vi "ex_3_testy.vi"() -> ()   [LabVIEW 2020]
panel:
  out "XY Graph 4":cluster{i32[], i32[]}(graph)
  out "XY Graph 3":cluster{i32[], i32[]}(graph)
  out "XY Graph 2":cluster{i32[], i32[]}(graph)
  out "XY Graph":cluster{i32[], i32[]}[](graph)
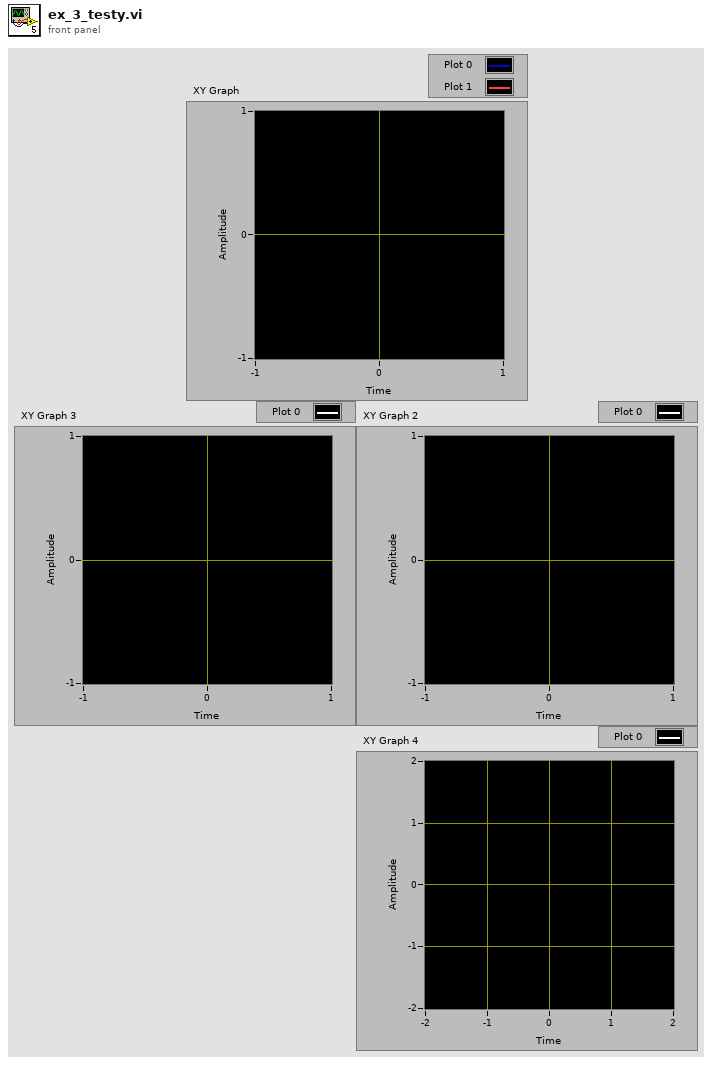
[diagram p1: front panel]
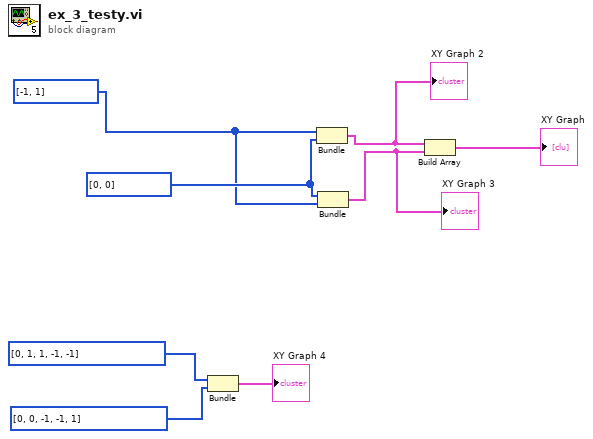
[diagram p0: block diagram]
diagram:
  w5 = i32[] [0, 0]
  w4 = i32[] [-1, 1]
  n1 = Bundle(i32[] [0, 1, 1, -1, -1], i32[] [0, 0, -1, -1, 1]) -> (→"XY Graph 4":cluster{i32[], i32[]})  [unwired: 1 in]
  n2 = Bundle(w4, w5) -> (w7:cluster{i32[], i32[]})  [unwired: 1 in]
  "XY Graph 2" <- w7
  n3 = Bundle(w5, w4) -> (w6:cluster{i32[], i32[]})  [unwired: 1 in]
  "XY Graph 3" <- w6
  n4 = Build Array(w7, w6) -> (→"XY Graph":cluster{i32[], i32[]}[])
